vi "onProcessStarted.vi"(8 "error in (no error)":errorcluster, 11 "CircularBuffer":refnum<class "CircularBuffer.lvclass">) -> (0 "error out":errorcluster, 3 "CircularBuffer out":refnum<class "CircularBuffer.lvclass">)   [LabVIEW 2013, in "CircularBuffer.lvclass"]
doc: "JKI State Machine Objects (SMO) 1.0.4.18\nJKI - JKI\nCopyright (c) 2016, JKI"
uses:
  CircularBuffer.lvclass
  <vilib>/JKI/JKI SMO/SMO/SMO.lvclass
panel:
  # "For instructions on how to use the JKI State Machine Objects, examples and video tutorials, visit:\nhttp://jki.net/state-machine-objects/\n\nJKI State Machine Objects™\nhttp://jki.net/state-machine-objects/\nCopyright (C) 2005-2015, JKI <info@jki.net>\nALL RIGHTS RESERVED"
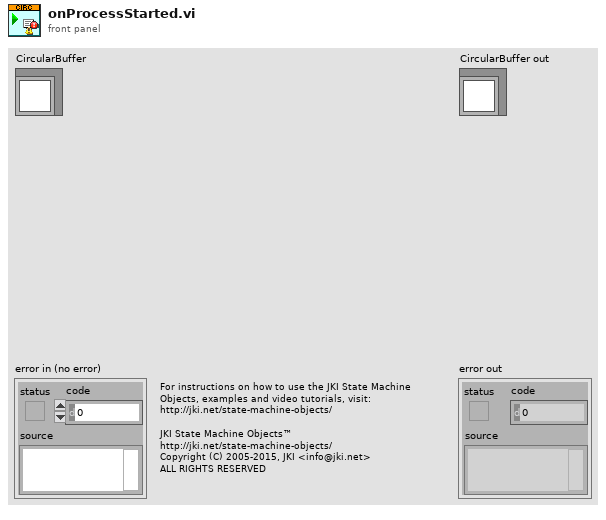
[diagram p1: front panel]
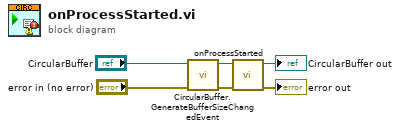
[diagram p0: block diagram]
diagram:
  n1 = call "CircularBuffer.GenerateBufferSizeChangedEvent.vi"("error in (no error)"="error in (no error)", "CircularBuffer in"="CircularBuffer") -> ("error out"=w3:errorcluster, "CircularBuffer out"=w4:refnum<class "CircularBuffer.lvclass">)  [unwired: 8 in]
  n2 = call-parent "onProcessStarted.vi"("error in (no error)"=w3, "SMO"=w4) -> ("error out"=→"error out":errorcluster, "SMO out"=→"CircularBuffer out":refnum<class "CircularBuffer.lvclass">)  [unwired: 8 in]
